vi "citTemplate.writeQueueWithAck.vi"(0 "timeout ms (-1)":i32=-1, 1 "High priority (F)":bool, 2 "instance (0)":i32, 3 "timeout error code (5003)":i32=5003, 5 "event in":variant, 9 "(flatten) data in":string, 11 "error in (no error)":errorcluster) -> (6 "dup of event":variant, 10 "notification data":string, 15 "error out":errorcluster)   [LabVIEW 2016]
uses:
  citTemplate.eventQueue.ctl
  citTemplate.queueData.ctl
  citTemplate.notifierHandle.ctl
  citTemplate.notifierData.ctl
panel:
  # "REENTRANT !!!!"
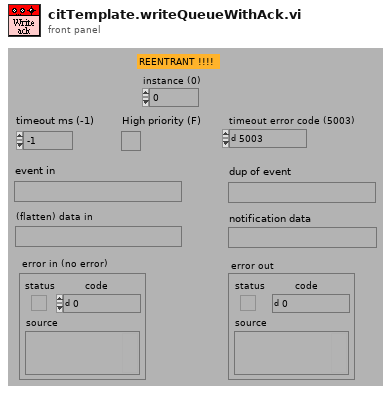
[diagram p1: front panel]
types:
  T1 = typedef "citTemplate.notifierData.ctl" = cluster{"notification data":string, "error":errorcluster}
  T2 = typedef "citTemplate.queueData.ctl" = cluster{"event index":u32, "(flatten) data in":string, "notifierHandle":T3}
  T3 = typedef "citTemplate.notifierHandle.ctl" = refnum<notifier>
  T4 = typedef "citTemplate.eventQueue.ctl" = enum16{"create queue", "get queue handle(s)", "destroy queue"}
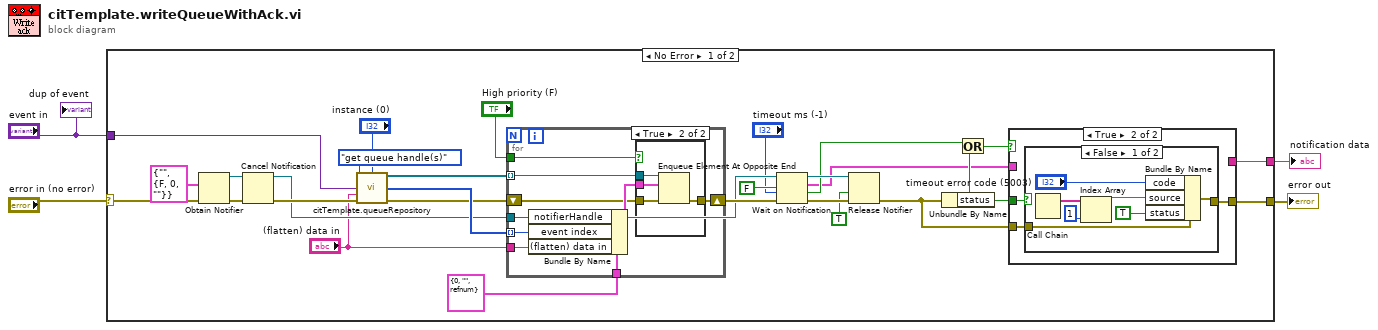
[diagram p0: block diagram]
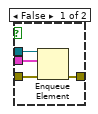
[diagram p2: hidden frame]
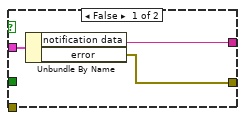
[diagram p3: hidden frame]
diagram:
  n1 = case shown="No Error" "error in (no error)" {
    selector: "error in (no error)" -> [w17 w64]
    tunnel: [w32 w64] -> w4
    tunnel: "event in" -> [w15 _]
    tunnel: [w9 _] -> w1
    frame No Error {
      n2 = Obtain Notifier(notification data type=T1 {"notification data"="", "error"={"status"=FALSE, "code"=0, "source"=""}} ("notifierData"), error in (no error)=w17) -> (notifier out=w16:refnum<notifier>, error out=w28:errorcluster)  [unwired: 1 in, 2 out]
      n3 = Cancel Notification(0:w16, 3:w28) -> (8:w14:refnum<notifier>, 11:w18:errorcluster)  [unwired: 1 out]
      n4 = call "citTemplate.queueRepository.vi"("mode (get queue handle)"=citTemplate.eventQueue."get queue handle(s)" ("mode (write event)"), "instance (0)"="instance (0)", "event in"=w15, "(flatten) data in"="(flatten) data in", "error in (no error)"=w18) -> ("queueHandle(s) out"=w27:refnum<queue>[], "eventIndex(s)"=w26:u32[], "error out"=w25:errorcluster)  [unwired: 3 in, 5 out]
      n5 = for {
        tunnel: w27 -> [w41] mode=indexing
        tunnel: "(flatten) data in" -> [w39]
        tunnel: "High priority (F)" -> [w38]
        tunnel: w14 -> [w37]
        tunnel: w26 -> [w36] mode=indexing
        shift-right: [w34] -> w24
        shift-left: w25 -> [w35]
        tunnel: T2 {"event index"=0, "(flatten) data in"="", "notifierHandle"=refnum} ("queueData") -> [w33]
        n6 = Bundle By Name(cluster=w33, "notifierHandle"=w37, "event index"=w36, "(flatten) data in"=w39) -> (w40:T2)
        n7 = case shown="True" w38 {
          tunnel: w41 -> [w45 w49]
          tunnel: w35 -> [w44 w48]
          tunnel: [w43 w47] -> w34
          tunnel: w40 -> [w42 w46]
          frame False {
            n8 = Enqueue Element(queue=w45, element=w42, error in (no error)=w44) -> (error out=w43:errorcluster)  [unwired: 3 out]
          }
          frame True {
            n9 = Enqueue Element At Opposite End(queue=w49, element=w46, error in (no error)=w48) -> (error out=w47:errorcluster)  [unwired: 3 out]
          }
        }
      }
      n10 = Wait on Notification(notifier=w14, ignore previous (F)=FALSE ("ignore previous (T)"), timeout in ms (-1)="timeout ms (-1)", error in (no error)=w24) -> (notifier out=w21:refnum<notifier>, notification=w10:T1, timed out?=w11:bool, error out=w20:errorcluster)
      n11 = Release Notifier(notifier=w21, force destroy? (F)=TRUE, error in (no error)=w20) -> (error out=w12:errorcluster)  [unwired: 2 out]
      n12 = Unbundle By Name(w12) -> ("status"=w29:bool)
      n13 = Or(x=w11, y=w29) -> (x .or. y?=w30:bool)
      n14 = case shown="True" w30 {
        tunnel: w10 -> [w52 _]
        tunnel: [w51 w53] -> w32
        tunnel: w12 -> [_ w55]
        tunnel: w29 -> [_ w54]
        tunnel: [w50 _] -> w9
        frame False {
          n15 = Unbundle By Name(w52) -> ("notification data"=w50:string, "error"=w51:errorcluster)
        }
        frame True {
          n16 = case shown="False" w54 {
            tunnel: w55 -> [w62 w63]
            tunnel: [w61 w63] -> w53
            frame False {
              n17 = Call Chain() -> (call chain=w58:string[])
              n18 = Index Array(array=w58, index=1) -> (element=w57:string)
              n19 = Bundle By Name(cluster=w62, "code"="timeout error code (5003)", "source"=w57, "status"=TRUE) -> (w61:errorcluster)
            }
            frame True {
            }
          }
        }
      }
    }
    frame Error {
    }
  }
  "error out" <- w4
  "notification data" <- w1
  "dup of event" <- "event in"
